vi "Configure SPI.vi"(5 "Purpose (\"SPI\")":string="SPI", 6 "SPI Config":T1={"Mode"=0, "Data Bits"=8, "Pins"={"TX GPIO"=7, "RX GPIO"=4, "SCK GPIO"=6}}, 7 "SPI #":T5=-1, 8 "error in (no error)":errorcluster, 10 "Baud":u32=1000000 format="%.0p", 11 "Session in":refnum<class "Session.lvclass">) -> (0 "error out":errorcluster, 3 "Session out":refnum<class "Session.lvclass">)   [LabVIEW 2024, in "CTI.lvlib" / "Session.lvclass"]
doc: "SPI (Serial Peripheral Interface) is a common communication bus for interacting with numerous sensors, displays, and other peripherals. SPI works by simultaneously transmitting and reading data for specific peripherals. Several peripherals can share the same data lines and are typically signalled by a \"CS\" gpio signal so the peripheral knows it should interact with the bus. For coordinated operations using a CS signal, check out the <b>SPI Communication.lvclass</b>."
uses:
  Session.lvclass
  SPI Number.ctl
  SPI Config.ctl
  SPI Mode.ctl
  SPI Pins.ctl
  GPIO Number.ctl
  Session.lvclass/Session.ctl
  7e7b61e7-8264-4332-8aa7-581be85c5de9.vi
  Is Full Errors.vi
  Check Errors.vi
  CTI.lvlib
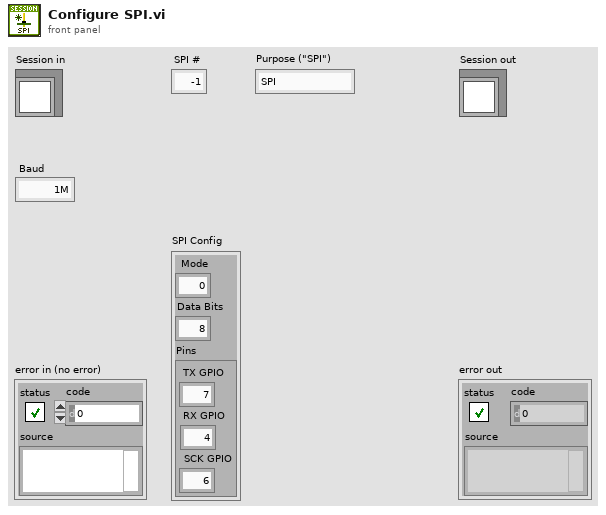
[diagram p1: front panel]
types:
  T1 = typedef "CTI.lvlib/SPI Config.ctl" = cluster{"Mode":T2, "Data Bits":i8, "Pins":T3}
  T2 = typedef "CTI.lvlib/SPI Mode.ctl" = i8
  T3 = typedef "CTI.lvlib/SPI Pins.ctl" = cluster{"TX GPIO":T4, "RX GPIO":T4, "SCK GPIO":T4}
  T4 = typedef "CTI.lvlib/GPIO Number.ctl" = i8
  T5 = typedef "CTI.lvlib/SPI Number.ctl" = i8
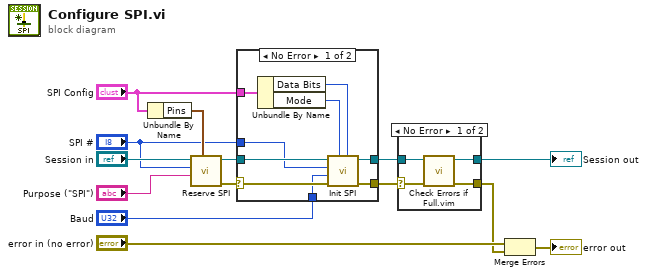
[diagram p0: block diagram]
diagram:
  n1 = Unbundle By Name("SPI Config") -> ("Pins"=w12:T3)
  n2 = call "Reserve SPI.vi"("SPI Pins"=w12, "Purpose"="Purpose (\"SPI\")", "SPI #"="SPI #", "Session in"="Session in") -> ("error out"=w10:errorcluster, "Session out"=w9:refnum<class "Session.lvclass">)  [unwired: 6 in]
  n3 = case shown="No Error" w10 {
    selector: w10 -> [w22 w24]
    tunnel: w9 -> [w23 w25]
    tunnel: "SPI Config" -> [w21 _]
    tunnel: "Baud" -> [w18 _]
    tunnel: [w17 w24] -> w5
    tunnel: [w16 w25] -> w6
    tunnel: "SPI #" -> [w15 _]
    frame No Error {
      n4 = Unbundle By Name(w21) -> ("Data Bits"=w19:i8, "Mode"=w20:T2)
      n5 = call "Init SPI.vi"("Data Bits"=w19, "Mode"=w20, "error in (no error)"=w22, "Baud"=w18, "SPI #"=w15, "Session in"=w23) -> ("error out"=w17:errorcluster, "Session out"=w16:refnum<class "Session.lvclass">)  [unwired: 4 in]
    }
    frame Error {
    }
  }
  n6 = case shown="No Error" w5 {
    selector: w5 -> [w28 w31]
    tunnel: w6 -> [w29 w30]
    tunnel: [w27 w30] -> w4
    tunnel: [w26 w31] -> w2
    frame No Error {
      n7 = call "Check Errors if Full.vim"("error in (no error)"=w28, "Session in"=w29) -> ("error out"=w26:errorcluster, "Session out"=w27:refnum<class "Session.lvclass">)  [unwired: 8 in]
    }
    frame Error {
    }
  }
  "Session out" <- w4
  n8 = Merge Errors("error in (no error)", w2) -> (→"error out":errorcluster)
